vi "Turret_Hardware_Globals.vi"() -> ()   [LabVIEW 2020]
panel:
  in  "Turret_Ref":string="Turret_Ref"
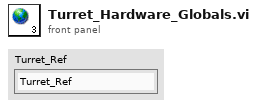
[diagram p1: front panel]
diagram:
